vi "Configure Modulation (Pulse Width).vi"(0 "VISA resource name":refnum<visa-resource-name>, 1 "Modulation Frequency (100.00 Hz)":dbl=100.0 min=0.002 max=20000.0 format="%.2f", 2 "Pulse Width Deviation (10e-6 s)":dbl=1e-05 min=0.0 max=100.0 format="%#.9g", 3 "Duty Cycle Deviation (0 %)":dbl min=0.0 max=100.0 format="%.2f", 5 "Enable Pulse Width Modulation (T: Enable)":bool=TRUE, 7 "Pulse Width Modulation Source (0: Internal)":u16(ring) items=["Internal", "External"], 9 "Modulation Waveform (0: Sine)":i32(ring) items=["Sine", "Square", "Ramp", "Negative Ramp", "Triangle", "Noise", "Arbitrary Waveform"], 11 "error in (no error)":errorcluster) -> (4 "VISA resource name out":refnum<visa-resource-name>, 15 "error out":errorcluster)   [LabVIEW 2012, in "Agilent 33XXX Series.lvlib"]
doc: "Allows and configures pulse width modulation. The width of a pulse waveform is varied by the instantaneous voltage of the modulating waveform.\n\nNote:\n(1) This VI is only used with the Agilent 33210A and 33220A.\n(2) The selected waveform must be Pulse.\n(3) Before using this mode, all other modes must be turned off."
uses:
  <instrlib>/Agilent 33XXX Series/Agilent 33XXX Series.lvlib
panel:
  # "Internal Pulse Width Modulation Settings"
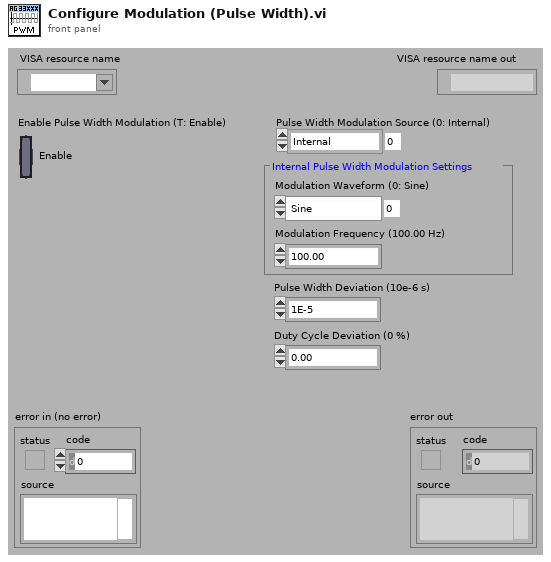
[diagram p1: front panel]
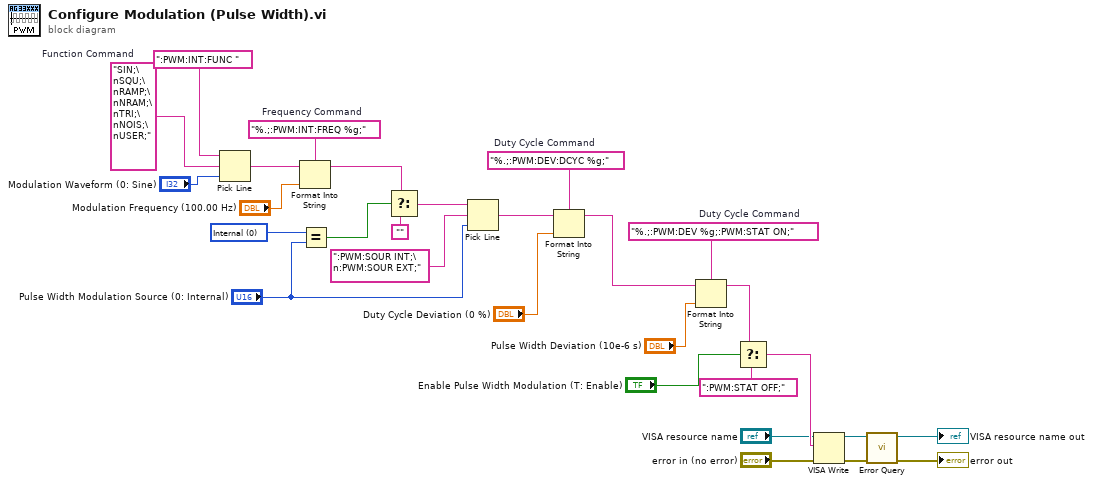
[diagram p0: block diagram]
diagram:
  w17 = "SIN;\nSQU;\nRAMP;\nNRAM;\nTRI;\nNOIS;\nUSER;"  # Function Command
  w19 = "%.;:PWM:INT:FREQ %g;"  # Frequency Command
  w20 = "%.;:PWM:DEV %g;:PWM:STAT ON;"  # Duty Cycle Command
  w26 = "%.;:PWM:DEV:DCYC %g;"  # Duty Cycle Command
  w11 = u16 0 items=["Internal", "External"] ("Source (0: Internal)")
  n1 = Pick Line(string ("")=":PWM:INT:FUNC ", multi-line string=w17, line index="Modulation Waveform (0: Sine)") -> (output string=w18:string)
  n2 = Format Into String(format string=w19, initial string=w18, "Modulation Frequency (100.00 Hz)") -> (resulting string=w15:string)  [unwired: 1 in, 1 out]
  n3 = Equal?(x=w11, y="Pulse Width Modulation Source (0: Internal)") -> (x = y?=w13:bool)
  n4 = Select(t=w15, s=w13, f="") -> (s? t:f=w12:string)
  n5 = Pick Line(string ("")=w12, multi-line string=":PWM:SOUR INT;\n:PWM:SOUR EXT;" ("Source Command"), line index="Pulse Width Modulation Source (0: Internal)") -> (output string=w9:string)
  n6 = Format Into String(format string=w26, initial string=w9, "Duty Cycle Deviation (0 %)") -> (resulting string=w21:string)  [unwired: 1 in, 1 out]
  n7 = Format Into String(format string=w20, initial string=w21, "Pulse Width Deviation (10e-6 s)") -> (resulting string=w8:string)  [unwired: 1 in, 1 out]
  n8 = Select(t=w8, s="Enable Pulse Width Modulation (T: Enable)", f=":PWM:STAT OFF;") -> (s? t:f=w6:string)
  n9 = VISA Write(VISA resource name="VISA resource name", write buffer=w6, error in (no error)="error in (no error)") -> (VISA resource name out=w29:refnum<visa-resource-name>, error out=w28:errorcluster)  [unwired: 1 out]
  n10 = call <instrlib>:"Error Query.vi"("error in (no error)"=w28, "VISA resource name"=w29) -> ("error out"=→"error out":errorcluster, "VISA resource name out"=→"VISA resource name out":refnum<visa-resource-name>)  [unwired: 6 in, 2 out]
